vi "SetUpE727.vi"(11 "stop":bool) -> (0 "Error Out":errorcluster, 1 "Redy":bool, 2 "Axis ID´s":string[](array[string]), 3 "SystemID":i32)   [LabVIEW 2019]
panel:
  out "Identification":string
  out "Configuration_Setup.vi is running":bool
  in  "Error In":errorcluster
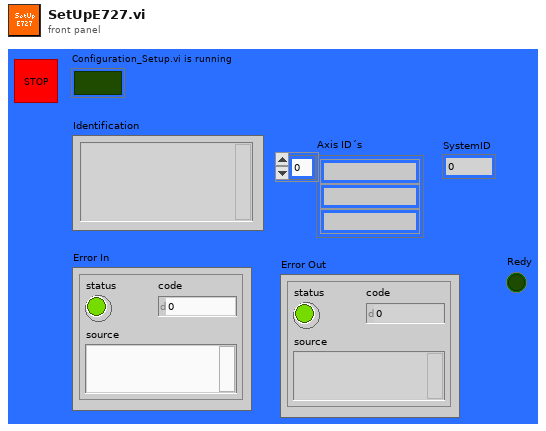
[diagram p1: front panel]
types:
  T1 = cluster{"Host address/name":string, "Port":i32, "Board":i32, "TCP/IP Search?":bool}
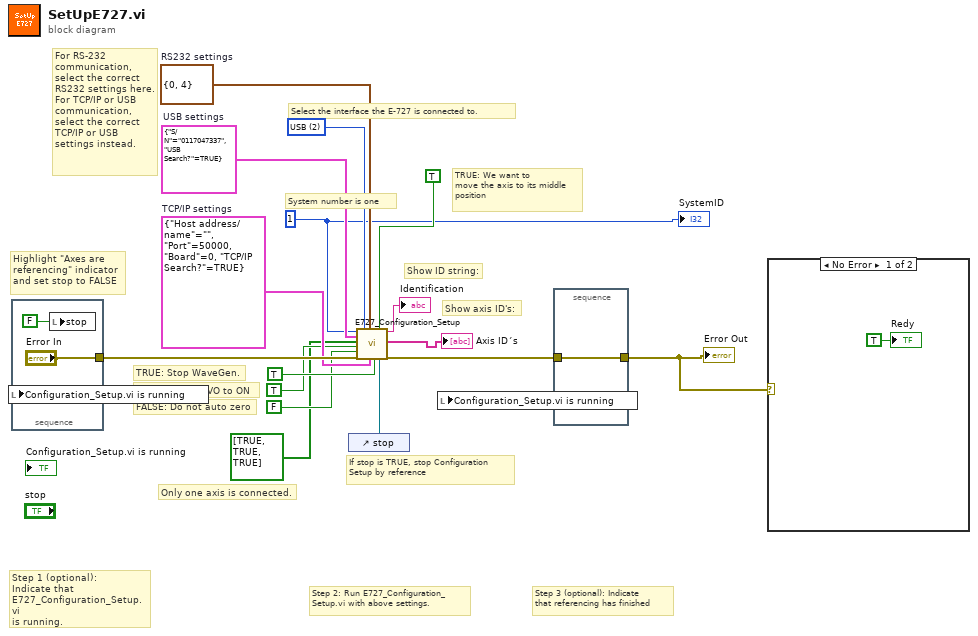
[diagram p0: block diagram]
diagram:
  w6 = cluster{"S/N":string, "USB Search?":bool} {"S/N"="0117047337", "USB Search?"=TRUE}  # USB settings
  w7 = u16 2 items=["RS232", "TCP/IP", "USB"] ("Interface")
  w9 = cluster{"Portnumber":i32, "Baudrate":u16} {"Portnumber"=0, "Baudrate"=4}  # RS232 settings
  w14 = T1 {"Host address/name"="", "Port"=50000, "Board"=0, "TCP/IP Search?"=TRUE}  # TCP/IP settings
  w2 = 1 ("System no.")
  # "Only one axis is connected."
  # "TRUE: We want to\nmove the axis to its middle\nposition"
  # "FALSE: Do not auto zero"
  # "TRUE: Switch SVO to ON"
  # "If stop is TRUE, stop Configuration\nSetup by reference"
  # "For RS-232 \ncommunication,\nselect the correct\nRS232 settings here.\nFor TCP/IP or USB \ncommunication, \nselect the correct \nTCP/IP or USB\nsettings instead."
  # "Select the interface the E-727 is connected to."
  # "Step 3 (optional): Indicate\nthat referencing has finished"
  # "Step 2: Run E727_Configuration_\nSetup.vi with above settings."
  # "Step 1 (optional): \nIndicate that\nE727_Configuration_Setup.vi\nis running."
  # "Highlight \"Axes are\nreferencing\" indicator\nand set stop to FALSE"
  # "Show axis ID's:"
  # "Show ID string:"
  # "TRUE: Stop WaveGen."
  # "System number is one"
  n1 = stacked-sequence {
    tunnel: ["Error In"] -> w15
    frame #0 {
      n2 = local write "Configuration_Setup.vi is running"(TRUE ("Configuration_Setup.vi is running")) -> ()
      n3 = local write "stop"(FALSE ("stop")) -> ()
    }
  }
  n4 = control-ref of="stop"() -> (w5:refnum<vi>)
  n5 = call "E727_Configuration_Setup.vi"("System no."=w2, "USB settings"=w6, "Are stages connected?"=bool[] [TRUE, TRUE, TRUE], "Change servo status to ON?"=TRUE ("Use dialog to define\nconnected stages?"), "Perform autozero?"=FALSE ("Use dialog to define\nconnected stages?"), "error in"=w15, "Interface"=w7, "RS232 settings"=w9, "TCP/IP settings"=w14, "Stop wave generator\noutput (if any)"=TRUE ("All axes?"), "Move to middle?"=TRUE, "Stop refnum"=w5) -> ("Identification"=→"Identification":string, "All conn. axes"=→"Axis ID´s":string[], "error out"=w16:errorcluster)  [unwired: 2 in, 3 out]
  n6 = stacked-sequence {
    tunnel: w16 -> [w21]
    tunnel: [w21] -> w1
    frame #0 {
      n7 = local write "Configuration_Setup.vi is running"(FALSE ("Configuration_Setup.vi is running")) -> ()
    }
  }
  "Error Out" <- w1
  n8 = case shown="No Error" w1 {
    frame No Error {
      "Redy" <- TRUE ("Redy")
    }
    frame Error {
    }
  }
  "SystemID" <- w2
